vi "Multiply.vi"(1 "B":T1={"Array Num"=[0, 0, 0, 0, 0, 0, 0, 0, 0, 0, 0, 0, 0, 0, 0, 0, 0, 0, 0, 0, 0, 0, 0, 0, 0, 0, 0, 0, 0, 0, 0, 0, 0, 0, 0, 0, 0, 0, 0, 0, 0, 0, 0, 0, 0, 0, 0, 0, 0, 0, 0, 0, 0, 0, 0, 0, 0, 0, 0, 0, 6, 5, 4, 5, 1, 5, 2, 8, 8, 3, 3, 7, 8, 2, 3, 2, 6, 1, 6, 8, 0, 0, 6, 8, 7, 8, 3, 9, 6, 7, 6, 7, 2, 5, 2, 1, 3, 4, 0, 3, 4, 4, 2, 8, 4, 2, 5, 4, 9, 6, 3, 4, 3, 1, 3, 2, 4, 0, 1, 6, 0, 3, 7, 8, 5, 3, 2, 4, 4, 0, 2, 9, 5, 0, 0, 5, 5, 7, 7, 1, 8, 2, 1, 8, 4, 7, 9, 0, 6, 0, 6, 3, 7, 9, 1, 0, 5, 3, 5, 5, 3, 4, 0, 7, 3, 9, 3, 7, 4, 7, 6, 9, 2, 5, 7, 9, 6, 0, 2, 1, 9, 2, 8, 3, 0, 1, 2, 7, 7, 5, 0, 2, 7, 0, 7, 5, 3, 9, 8, 3, 0, 2, 2, 2, 7, 9, 4, 9, 8, 4, 2, 4, 7, 8, 9, 1, 0, 3, 8, 9, 9, 8, 9, 2, 5, 2, 7, 7, 0, 0, 1, 9, 0, 5, 0, 8, 0, 5, 4, 5, 7, 3, 2, 9, 2, 3, 9, 4, 3, 9, 9, 8, 2, 9, 7, 7, 4, 0, 0, 1, 2, 7, 7, 7, 6, 3, 9, 0, 6, 3, 4, 8, 3, 2, 2, 2, 8, 3, 4, 0, 9, 4, 7, 9, 5, 4, 6, 7, 2, 2, 8, 4, 8, 5, 4, 4, 6, 0, 8, 0, 6, 8, 5, 4, 0, 3, 1, 1, 3, 4, 6, 1, 5, 1, 5, 6, 0, 9, 1, 7, 3, 8, 5, 9, 6, 0, 9, 1, 1, 7, 2, 7, 9, 6, 9, 2, 2, 1, 8, 3, 5, 0, 6, 8, 6, 7, 2, 5, 6, 3, 3, 5, 1, 1, 8, 2, 4, 3, 1, 2, 6, 3, 0, 8, 9, 6, 9, 0, 5, 9, 9, 4, 6, 3, 6, 0, 2, 7, 8, 8, 5, 9, 2, 8, 7, 3], "Decimal Index"=0, "stop"=FALSE}, 2 "A":T1={"Array Num"=[6, 1, 2, 9, 6, 5, 2, 6, 7, 9, 9, 2, 7, 8, 5, 9, 0, 2, 8, 5, 9, 4, 4, 3, 7, 3, 5, 6, 8, 1, 1, 4, 3, 0, 2, 6, 3, 3, 3, 7, 6, 8, 3, 7, 6, 0, 4, 7, 5, 9, 4, 4, 7, 5, 0, 5, 6, 7, 0, 8, 4, 6, 4, 4, 7, 8, 2, 4, 2, 4, 3, 0, 4, 1, 8, 2, 2, 7, 2, 1, 3, 6, 9, 9, 8, 9, 4, 1, 3, 2, 9, 4, 5, 4, 1, 8, 2, 4, 0, 4, 2, 9, 9, 1, 6, 8, 8, 2, 3, 3, 7, 2, 6, 8, 6, 4, 3, 8, 8, 7, 6, 6, 7, 6, 9, 6, 5, 0, 6, 3, 2, 8, 6, 3, 1, 3, 4, 8, 2, 0, 8, 4, 8, 8, 4, 4, 7, 1, 4, 0, 3, 5, 2, 9, 0, 2, 6, 2, 2, 8, 8, 0, 0, 6, 0, 0, 2, 3, 4, 3, 4, 9, 1, 9, 3, 8, 7, 3, 5, 1, 5, 4, 0, 7, 2, 1, 4, 0, 6, 8, 8, 8, 0, 3, 8, 0, 9, 8, 8, 4, 7, 6, 7, 5, 6, 5, 9, 2, 6, 9, 2, 4, 4, 8, 4, 4, 2, 3, 6, 4, 9, 9, 8, 0, 7, 5, 3, 9, 2, 2, 3, 0, 9, 3, 3, 4, 3, 9, 9, 4, 1, 0, 3, 0, 2, 9, 5, 5, 0, 0, 8, 0, 4, 7, 0, 9, 0, 6, 4, 9, 9, 1, 2, 4, 6, 9, 4, 0, 1, 2, 4, 3, 0, 8, 1, 9, 8, 9, 7, 8, 8, 8, 5, 3, 5, 3, 7, 2, 3, 6, 8, 4, 6, 9, 0, 1, 3, 5, 6, 6, 8, 1, 7, 1, 7, 4, 0, 0, 9, 5, 9, 9, 3, 2, 1, 5, 9, 6, 1, 9, 2, 4, 9, 2, 0, 3, 0, 4, 8, 5, 6, 8, 8, 9, 0, 4, 2, 5, 3, 9, 3, 3, 2, 9, 2, 1, 4, 0, 4, 4, 5, 3, 6, 4, 1, 0, 2, 0, 7, 5, 0, 0, 9, 7, 4, 0, 3, 3, 9, 0, 5, 2, 1, 0, 8, 6, 3, 9, 0, 0, 9, 3, 0, 3, 9, 2, 3, 4, 5, 6, 7, 1, 2, 2, 1, 8, 5, 9, 8, 7, 7, 1, 5, 9, 0, 6, 9, 8, 7, 3, 4, 8, 9, 9, 7, 9, 1, 1, 0, 7, 8, 1, 8, 5, 9, 9, 6, 7, 6, 5, 8, 3, 1, 5, 6, 7, 1, 4, 5, 7, 8, 8, 4, 8, 7, 9, 3, 7, 7, 4, 8, 9, 6, 4, 3, 7, 2, 8, 3, 5, 7, 2, 6, 5, 6, 6, 4, 4, 6, 6, 9, 7, 5, 4, 1, 8, 3, 1, 9, 3, 6, 8, 9, 4, 1, 8, 3, 2, 9, 1, 3, 3, 5, 9, 7, 2, 0, 7, 3, 3, 1, 9, 3, 5, 7, 1, 4, 4, 0, 9, 8, 1, 3, 9, 7, 9, 2, 0, 5, 9, 8, 2, 4, 6, 9, 1, 7, 3, 6, 0, 7, 6, 9, 8, 7, 1, 6, 4, 7, 1, 2, 9, 8, 1, 4, 4, 8, 3, 4, 7, 3, 7, 4, 6, 5, 2, 3, 0, 7, 8, 9, 1, 8, 0, 5, 9, 4, 7, 5, 0, 0, 9, 2, 2, 3, 8, 6, 9, 1, 3, 8, 9, 4, 7, 7, 8, 1, 0, 8, 4, 4, 1, 4, 9, 1, 5, 6, 6, 6, 9, 5, 4, 0, 2, 5, 4, 5, 1, 5, 5, 8, 5, 3, 7, 2, 7, 9, 1, 0, 0, 7, 5, 9, 9, 7, 1, 6, 9, 6, 5, 2, 1, 2, 9, 1, 6, 4, 7, 2, 5, 4, 4, 3, 6, 2, 0, 6, 7, 1, 7, 2, 6, 1, 3, 9, 0, 3, 6, 6, 7, 6, 8, 7, 2, 2, 3, 1, 7, 6, 8, 5, 5, 7, 7, 5, 4, 2, 2, 9, 5, 4, 8, 4, 7, 6, 6, 3, 0, 0, 5, 2, 7, 3, 4, 4, 8, 4, 8, 6, 1, 6, 8, 8, 1, 4, 7, 3], "Decimal Index"=0, "stop"=FALSE}) -> (0 "Answer":T1={"Array Num"=[1, 2, 3], "Decimal Index"=0, "stop"=FALSE})   [LabVIEW 2025]
uses:
  Number.ctl
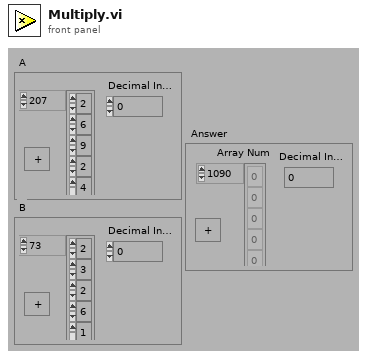
[diagram p1: front panel]
types:
  T1 = typedef "Number.ctl" = cluster{"Array Num":i8[], "Decimal Index":i32, "stop":bool}
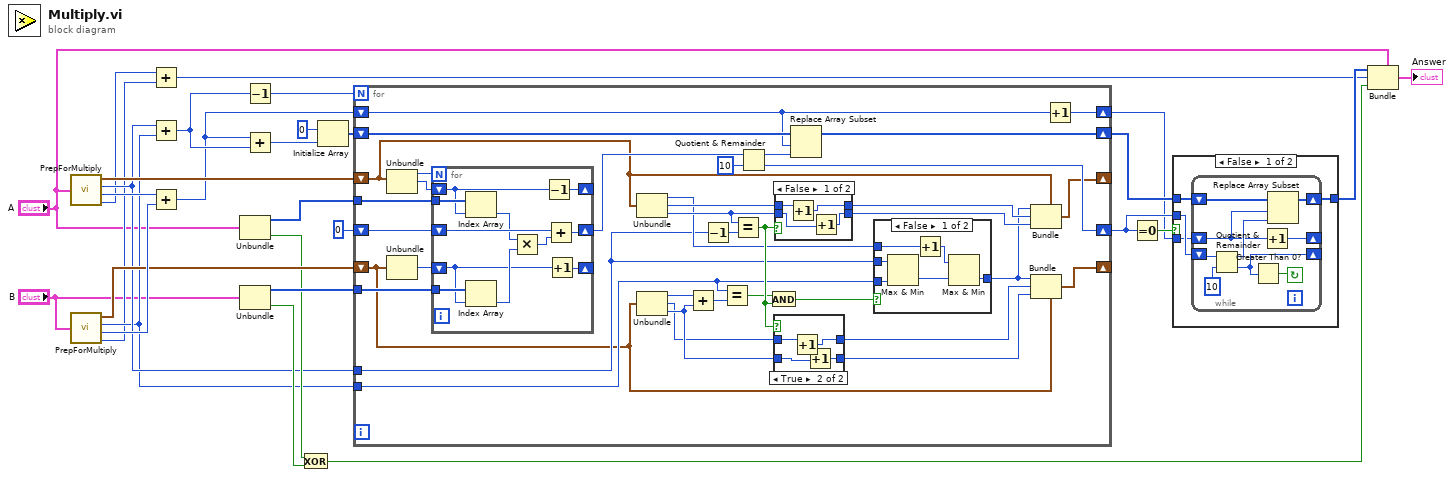
[diagram p0: block diagram]
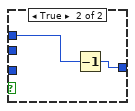
[diagram p5: hidden frame]
diagram:
  n1 = call "PrepForMultiply.vi"("A"="A") -> ("Starting Condition"=w20:cluster{"digit":i32, i32, i32}, "Working Digits"=w16:i32, "Trailing Zeroes"=w28:i32, "New Decimal Index"=w10:i32)
  n2 = call "PrepForMultiply.vi"("A"="B") -> ("Starting Condition"=w21:cluster{"digit":i32, i32, i32}, "Working Digits"=w15:i32, "Trailing Zeroes"=w27:i32, "New Decimal Index"=w9:i32)
  n3 = Add(x=w10, y=w9) -> (x+y=w8:i32)
  n4 = Add(x=w16, y=w15) -> (x+y=w7:i32)
  n5 = Add(x=w28, y=w27) -> (x+y=w4:i32)
  n6 = Unbundle("A") -> ("Array Num"=w25:i8[], "stop"=w19:bool)  [unwired: 1 out]
  n7 = Unbundle("B") -> ("Array Num"=w24:i8[], "stop"=w18:bool)  [unwired: 1 out]
  n8 = Decrement(x=w7) -> (x-1=w26:i32)
  n9 = Add(x=w4, y=w7) -> (x+y=w6:i32)
  n10 = Exclusive Or(1:w18, 2:w19) -> (0:w17:bool)
  n11 = Initialize Array(i8 0 ("digit"), w6) -> (w23:i8[])
  n12 = for {
    N: w26 -> [_]
    shift-right: [w62] -> w13
    shift-left: w23 -> [w63]
    shift-right: [w34] -> _
    shift-left: w20 -> [w37]
    shift-right: [w33] -> _
    shift-left: w21 -> [w30]
    tunnel: w25 -> [w65]
    tunnel: w24 -> [w64]
    shift-right: [w58] -> w14
    shift-left: 0 ("digit 2") -> [w61]
    tunnel: w16 -> [w36]
    tunnel: w15 -> [w35]
    shift-right: [w32] -> w3
    shift-left: w4 -> [w31]
    n13 = Unbundle(w37) -> ("digit"=w56:i32, w55:i32)  [unwired: 1 out]
    n14 = Unbundle(w30) -> (w54:i32)  [unwired: 2 out]
    n15 = for {
      N: w56 -> [_]
      tunnel: w65 -> [w96]
      tunnel: w64 -> [w95]
      shift-right: [w93] -> w60
      shift-left: w61 -> [w94]
      shift-right: [w89] -> _
      shift-left: w55 -> [w88]
      shift-right: [w87] -> _
      shift-left: w54 -> [w86]
      n16 = Index Array(array=w96, index=w88) -> (element=w90:i8)
      n17 = Index Array(array=w95, index=w86) -> (element=w91:i8)
      n18 = Multiply(x=w90, y=w91) -> (x*y=w92:i8)
      n19 = Decrement(x=w88) -> (x-1=w89:i32)
      n20 = Add(x=w94, y=w92) -> (x+y=w93:i32)
      n21 = Increment(x=w86) -> (x+1=w87:i32)
    }
    n22 = Unbundle(w37) -> ("digit"=w38:i32, w45:i32, w47:i32)
    n23 = Unbundle(w30) -> ("digit"=w40:i32, w50:i32, w53:i32)
    n24 = Add(x=w40, y=w53) -> (x+y=w42:i32)
    n25 = Decrement(x=w36) -> (x-1=w44:i32)
    n26 = Equal?(x=w35, y=w42) -> (x = y?=w43:bool)
    n27 = Equal?(x=w47, y=w44) -> (x = y?=w49:bool)
    n28 = Quotient & Remainder(x=w60, y=10 ("digit 2")) -> (x-y*floor(x/y)=w57:i32, floor(x/y)=w58:i32)
    n29 = And(x=w43, y=w49) -> (x .and. y?=w41:bool)
    n30 = case shown="True" w49 {
      tunnel: w50 -> [w67 w71]
      tunnel: [w67 w70] -> w51
      tunnel: w53 -> [w66 w69]
      tunnel: [w66 w68] -> w52
      frame False {
      }
      frame True {
        n31 = Increment(x=w71) -> (x+1=w70:i32)
        n32 = Increment(x=w69) -> (x+1=w68:i32)
      }
    }
    n33 = case shown="False" w49 {
      tunnel: w45 -> [w75 w77]
      tunnel: [w74 w77] -> w46
      tunnel: w47 -> [w73 w76]
      tunnel: [w72 w76] -> w48
      frame False {
        n34 = Increment(x=w75) -> (x+1=w74:i32)
        n35 = Increment(x=w73) -> (x+1=w72:i32)
      }
      frame True {
      }
    }
    n36 = Replace Array Subset(array=w63, new element=w57, index=w31) -> (w62:i8[])
    n37 = case shown="False" w41 {
      tunnel: w38 -> [w82 w85]
      tunnel: w35 -> [w81 _]
      tunnel: w36 -> [w79 _]
      tunnel: [w78 w84] -> w39
      frame False {
        n38 = Max & Min(x=w79, y=w81) -> (min(x,y)=w80:i32)  [unwired: 1 out]
        n39 = Increment(x=w82) -> (x+1=w83:i32)
        n40 = Max & Min(x=w83, y=w80) -> (min(x,y)=w78:i32)  [unwired: 1 out]
      }
      frame True {
        n41 = Decrement(x=w85) -> (x-1=w84:i32)
      }
    }
    n42 = Bundle(cluster=w37, "digit"=w39, w46, w48) -> (w34:cluster{"digit":i32, i32, i32})
    n43 = Bundle(cluster=w30, "digit"=w39, w51, w52) -> (w33:cluster{"digit":i32, i32, i32})
    n44 = Increment(x=w31) -> (x+1=w32:i32)
  }
  n45 = Equal To 0?(x=w14) -> (x = 0?=w11:bool)
  n46 = case shown="False" w11 {
    tunnel: w13 -> [w100 w110]
    tunnel: [w99 w110] -> w12
    tunnel: w14 -> [w98 _]
    tunnel: w3 -> [w97 _]
    frame False {
      n47 = while {
        shift-left: w98 -> [w108]
        shift-right: [w106] -> _
        shift-right: [w103] -> w99
        shift-left: w100 -> [w104]
        shift-right: [w102] -> _
        shift-left: w97 -> [w101]
        stop <- w107 continue-if-true
        n48 = Quotient & Remainder(x=w108, y=10) -> (x-y*floor(x/y)=w105:i32, floor(x/y)=w106:i32)
        n49 = Greater Than 0?(x=w106) -> (x > 0?=w107:bool)
        n50 = Increment(x=w101) -> (x+1=w102:i32)
        n51 = Replace Array Subset(array=w104, new element=w105, index=w101) -> (w103:i8[])
      }
    }
    frame True {
    }
  }
  n52 = Bundle(cluster="A", "Array Num"=w12, "Decimal Index"=w8, "stop"=w17) -> (→"Answer":T1)
